vi "Read Roles.vi"(8 "error in (no error)":errorcluster, 11 "5RobotsPassGamePlay in":refnum<class "5RobotsPassGamePlay.lvclass">) -> (0 "error out":errorcluster, 2 "Roles":T1, 3 "5RobotsPassGamePlay out":refnum<class "5RobotsPassGamePlay.lvclass">)   [LabVIEW 2023, in "5RobotsPassGamePlay.lvclass"]
uses:
  5RobotsPassGamePlay.lvclass
  PassBestRobotRole_class/PassBestRobotRole.lvclass
  5RobotsRole_class/5RobotsRole.lvclass
  PassBestReceiverRole_class/PassBestReceiverRole.lvclass
  5RobotsPassGamePlay.lvclass/5RobotsPassGamePlay.ctl
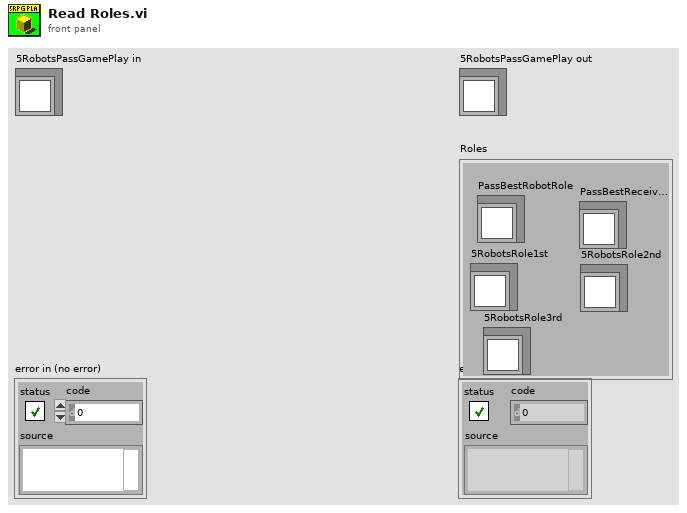
[diagram p1: front panel]
types:
  T1 = cluster{"PassBestRobotRole":refnum<class "PassBestRobotRole.lvclass">, "5RobotsRole3rd":refnum<class "5RobotsRole.lvclass">, "5RobotsRole2nd":refnum<class "5RobotsRole.lvclass">, "5RobotsRole1st":refnum<class "5RobotsRole.lvclass">, "PassBestReceiverRole":refnum<class "PassBestReceiverRole.lvclass">}
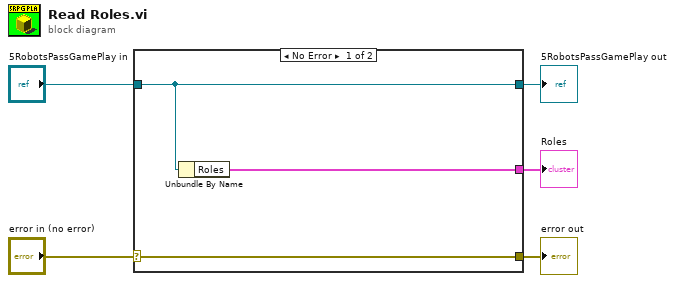
[diagram p0: block diagram]
diagram:
  n1 = case shown="No Error" "error in (no error)" {
    selector: "error in (no error)" -> [w8 w9]
    tunnel: [w8 w9] -> w4
    tunnel: [w7 w10] -> w2
    tunnel: "5RobotsPassGamePlay in" -> [w7 w10]
    tunnel: [w6 _] -> w1
    frame No Error {
      n2 = Unbundle By Name(w7) -> ("Roles"=w6:T1)
    }
    frame Error {
    }
  }
  "error out" <- w4
  "5RobotsPassGamePlay out" <- w2
  "Roles" <- w1
